vi "写入VISA resource name.vi"(8 "error in (no error)":errorcluster caption="错误输入（无错误）", 10 "VISA resource name":refnum<visa-resource-name>, 11 "DMM输入":refnum<class "DMM.lvclass">) -> (0 "error out":errorcluster caption="错误输出", 3 "DMM输出":refnum<class "DMM.lvclass">)   [LabVIEW 2020, in "DMM.lvlib" / "DMM.lvclass"]
uses:
  DMM.lvclass
  DMM.lvclass/DMM.ctl
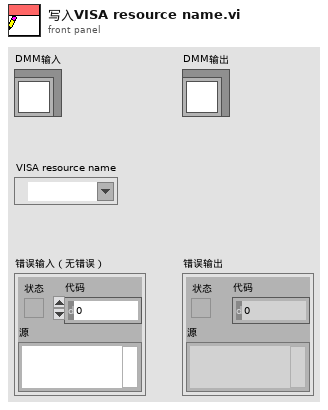
[diagram p1: front panel]
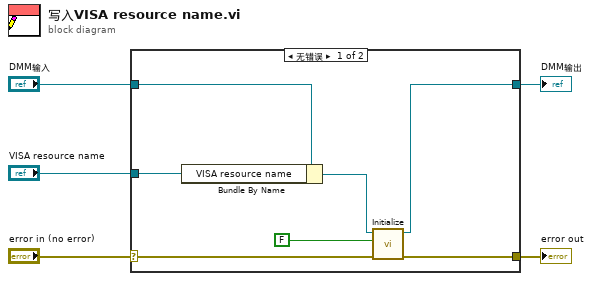
[diagram p0: block diagram]
diagram:
  n1 = case shown="无错误" "error in (no error)" {
    selector: "error in (no error)" -> [w10 w13]
    tunnel: [w9 w13] -> w4
    tunnel: [w7 w14] -> w2
    tunnel: "DMM输入" -> [w12 w14]
    tunnel: "VISA resource name" -> [w11 _]
    frame No Error {
      n2 = Bundle By Name(cluster=w12, "VISA resource name"=w11) -> (w8:refnum<class "DMM.lvclass">)
      n3 = call-dynamic "Initialize.vi"("error in (no error)"=w10, "Reset? (T: Reset)"=FALSE, "DMM 输入"=w8) -> ("error out"=w9:errorcluster, "DMM 输出"=w7:refnum<class "DMM.lvclass">)  [unwired: 7 in]
    }
    frame Error {
    }
  }
  "error out" <- w4
  "DMM输出" <- w2
